vi "GUI Measurement setup.vi"(11 "Measurement properties":T3={"Measurement ID"=enum."1 signal, 1 ADC, 1 PJVS", "Description"="3 phase, 3 ADC, 1 PJVS", "Switching matrix M"=[], "Signal frequency  (Hz)"=50.0, "Maximal signal amplitude (V)"=0.0, "PRs (s)"=1.0, "PRe (s)"=10.0, "MRs (s)"=0.0, "MRe (s)"=0.0, "Set PJVS frequency (Hz)"=50.0, "PJVS reference voltages (1 period, V)"=[], "Requiested PJVS steps"=10, "Sampling f (Hz)"=0.0, "Trigger mode"=enum."Trigger every MX switch", "Timing matrix (periods)"=[], "Record length (multiples of M)"=1, "Calculated"={"Triggers to next path (line of sequence)"=[], "Record samples"=0, "Sample indexes of switches"=[], "PRs (samples)"=0, "PRe (samples)"=0, "MRs (samples)"=0, "MRe (samples)"=0, "Trigger frequency  (Hz)"=50.0, "Measurement druation (s)"=0.0, "Samples per step"=0.0, "QPMX Sequence"=[]}, "No of required digitizers"=0, "No of required transducers"=0, "Transducer correction files"=[], "Digitizer correction file"=path ""} {"Calculated"."Trigger frequency  (Hz)" format="%#_6p"; "Record length (multiples of M)" min=1 step=1; "PJVS reference voltages (1 period, V)" format="%.9g"; "MRe (s)" format="%#_4p"; "MRs (s)" format="%#_4p"; "PRe (s)" format="%#.4p"; "PRs (s)" format="%#_4p"}) -> (3 "Measurement properties out":T3={"Measurement ID"=enum."1 signal, 1 ADC, 1 PJVS", "Description"="3 phase, 3 ADC, 1 PJVS", "Switching matrix M"=[], "Signal frequency  (Hz)"=50.0, "Maximal signal amplitude (V)"=0.0, "PRs (s)"=1.0, "PRe (s)"=10.0, "MRs (s)"=0.0, "MRe (s)"=0.0, "Set PJVS frequency (Hz)"=50.0, "PJVS reference voltages (1 period, V)"=[], "Requiested PJVS steps"=10, "Sampling f (Hz)"=0.0, "Trigger mode"=enum."Trigger every MX switch", "Timing matrix (periods)"=[], "Record length (multiples of M)"=1, "Calculated"={"Triggers to next path (line of sequence)"=[], "Record samples"=0, "Sample indexes of switches"=[], "PRs (samples)"=0, "PRe (samples)"=0, "MRs (samples)"=0, "MRe (samples)"=0, "Trigger frequency  (Hz)"=50.0, "Measurement druation (s)"=0.0, "Samples per step"=0.0, "QPMX Sequence"=[]}, "No of required digitizers"=0, "No of required transducers"=0, "Transducer correction files"=[], "Digitizer correction file"=path ""} {"Calculated"."Trigger frequency  (Hz)" format="%#_6p"; "Record length (multiples of M)" min=1 step=1; "PJVS reference voltages (1 period, V)" format="%.9g"; "MRe (s)" format="%#_4p"; "MRs (s)" format="%#_4p"; "PRe (s)" format="%#.4p"; "PRs (s)" format="%#_4p"})   [LabVIEW 2020]
doc: "Use this template to build a producer/consumer design pattern with events to produce queue items. Use this design pattern instead of the User Interface Event Handler pattern for user interfaces when you want to execute code asynchronously in response to an event without slowing the user interface responsiveness."
uses:
  Measurement/Type definitions/Measuement properties.ctl
  Measurement/Type definitions/Measurement ID.ctl
  Measurement/Type definitions/Trigger mode.ctl
  <vilib>/Utility/error.llb/Error Cluster From Error Code.vi
  <vilib>/ErrorRing/Error Ring.xnode
  external libraries/varilib/varilib.lvlib
panel:
  in  "Digitizer correction file":path
  out "No of transducer corrections":u32=50 caption="Transducer corrections for           transducers."
  out "No of digitizer channels corrections":u32=50 caption="Corrections for           digitizer channels."
  in  "Transducer correction files":path[](array[path])
  out "required transducers":u32=50 caption="required."
  out "required digitizers":u32=50 caption="required."
  out "Connections image":picture
  out "Waveforms image":picture
  out "Samples per step":dbl
  out "Measurement druation (s)":dbl caption="Duration" format="%#_6p"
  in  "Maximal signal amplitude (V)":dbl caption="Maximal signal amplitude (at digitizer)"
  in  "Trigger mode":T1 caption="Mode"
  in  "Measurement setup ID":T2=enum."1 signal, 1 ADC, 1 PJVS" caption="Measurement scenario"
  out "Record samples":u32 format="%.0p"
  in  "Record length (multiples of M)":u32=1 min=1 step=1
  out "Trigger frequency  (Hz)":dbl=50.0 caption="Trigger frequency" format="%#_6p"
  in  "Sampling f (Hz)":dbl caption="Sampling frequency" format="%#_6p"
  in  "Requiested PJVS steps":u32=1 min=1 step=1
  in  "MRe (s)":dbl min=0.0 format="%#_4p"
  in  "MRs (s)":dbl min=0.0 format="%#_4p"
  in  "PRe (s)":dbl min=0.0 format="%#_4p"
  in  "PRs (s)":dbl min=0.0 format="%#_4p"
  in  "Signal frequency  (Hz)":dbl=50.0 caption="Signal frequency" format="%#_6p"
  out "Description":string
  out "gui_elements":refnum<vi>[](array[refnum])
  in  "save_and_quit":bool
  in  "cancel":bool
  # "Scenario"
  # "Signals"
  # "Hz"
  # "V"
  # "Sampling"
  # "Who will make\nnice pictures?\n\nconnection setup here"
  # "Hz"
  # "s"
  # "Trigger"
  # "Hz"
  # "PJVS"
  # "Who will make\nnice pictures?\n\nwaveforms here"
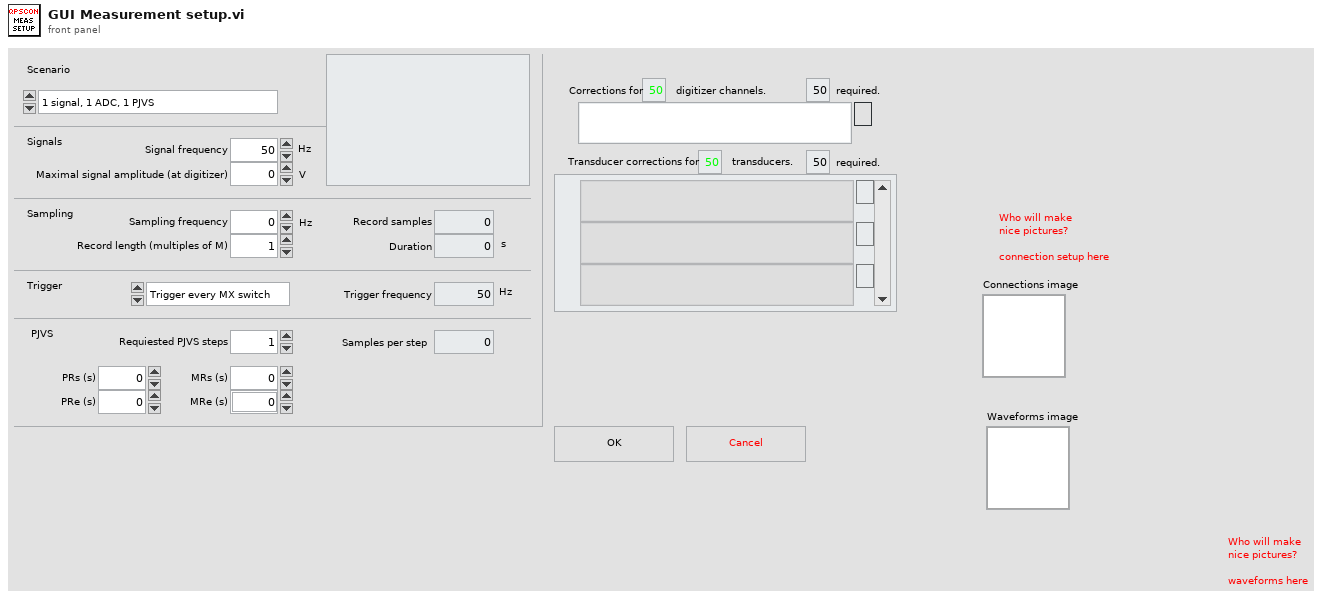
[diagram p1: front panel]
types:
  T1 = typedef "Trigger mode.ctl" = enum16{"Trigger every MX switch", "Trigger every sample"}
  T2 = typedef "Measurement ID.ctl" = enum16{"Manual setup", "1 signal, 1 ADC, 1 PJVS", "1 phase (U, I), 1 ADC, 1 PJVS", "1 phase (U, I), 2 ADC, 1 PJVS", "1 phase (U, I), 3 ADC, 1 PJVS", "3 phases (U1..3, I1..3), 3 ADC, 1 PJVS"}
  T3 = typedef "Measuement properties.ctl" = cluster{"Measurement ID":T2, "Description":string, "Switching matrix M":i32[][], "Signal frequency  (Hz)":dbl, "Maximal signal amplitude (V)":dbl, "PRs (s)":dbl, "PRe (s)":dbl, "MRs (s)":dbl, "MRe (s)":dbl, "Set PJVS frequency (Hz)":dbl, "PJVS reference voltages (1 period, V)":dbl[], "Requiested PJVS steps":u32, "Sampling f (Hz)":dbl, "Trigger mode":T1, "Timing matrix (periods)":i32[], "Record length (multiples of M)":u32, "Calculated":cluster{"Triggers to next path (line of sequence)":u32[], "Record samples":u32, "Sample indexes of switches":u32[], "PRs (samples)":i32, "PRe (samples)":i32, "MRs (samples)":i32, "MRe (samples)":i32, "Trigger frequency  (Hz)":dbl, "Measurement druation (s)":dbl, "Samples per step":dbl, "QPMX Sequence":bool[][]}, "No of required digitizers":u32, "No of required transducers":u32, "Transducer correction files":path[], "Digitizer correction file":path}
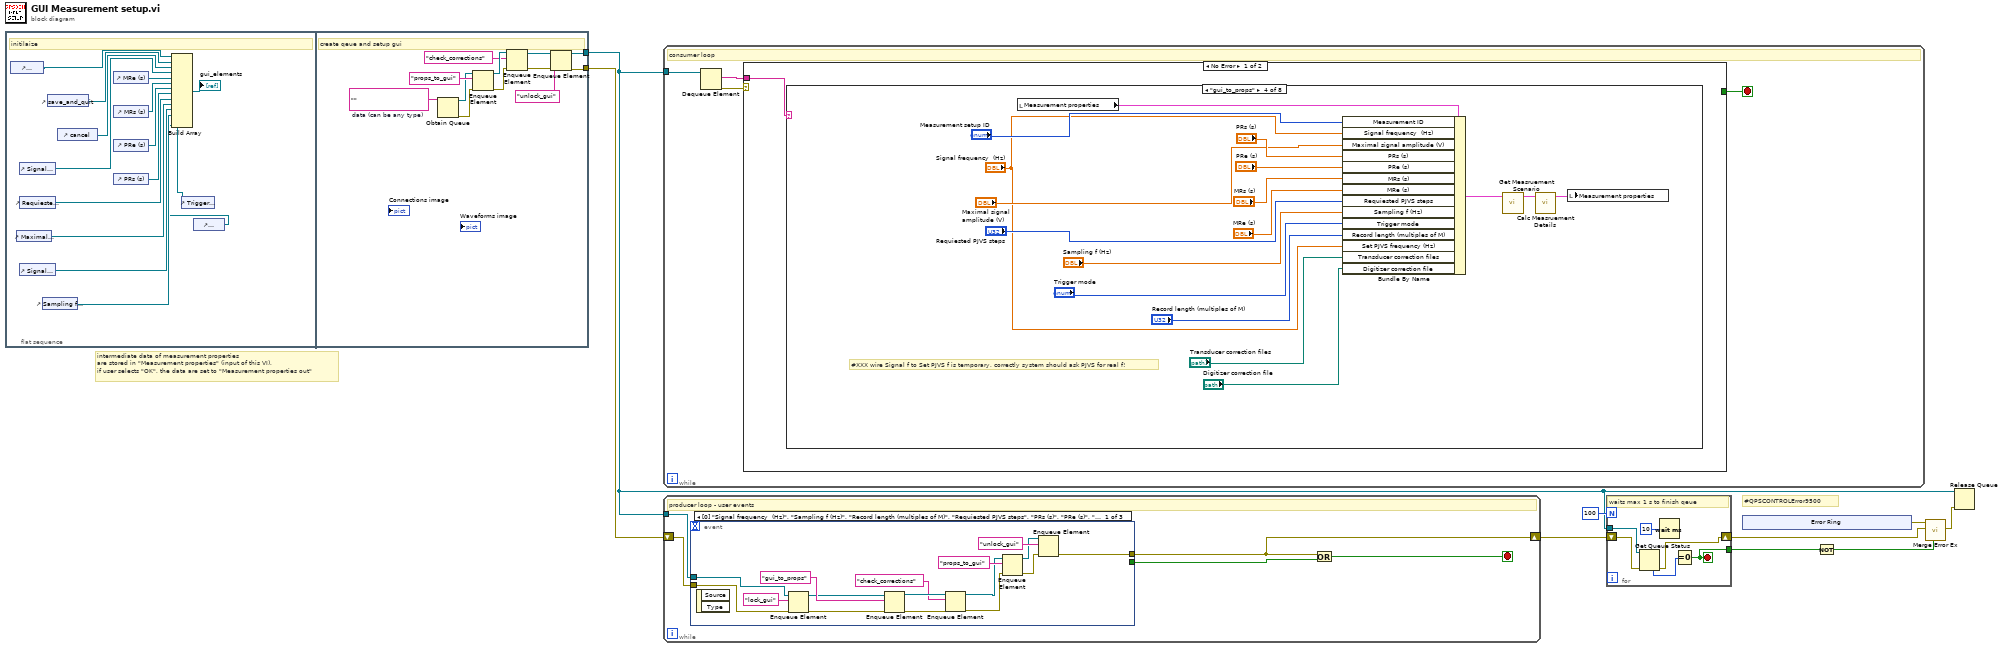
[diagram p0: block diagram]
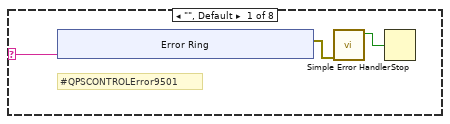
[diagram p2: hidden frame]
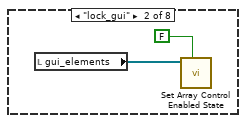
[diagram p3: hidden frame]
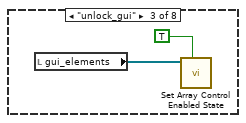
[diagram p4: hidden frame]
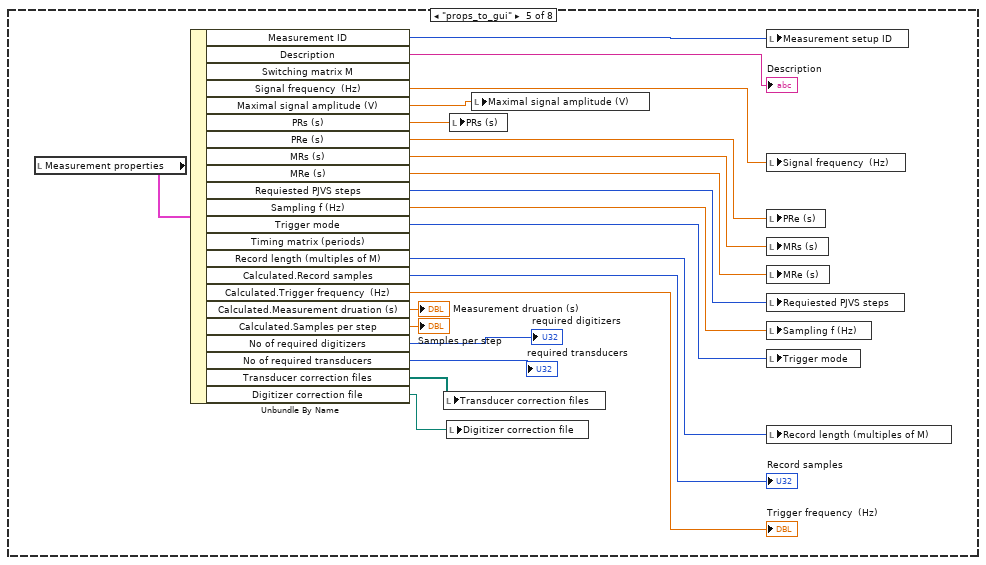
[diagram p5: hidden frame]
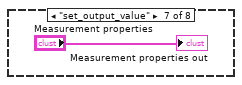
[diagram p7: hidden frame]
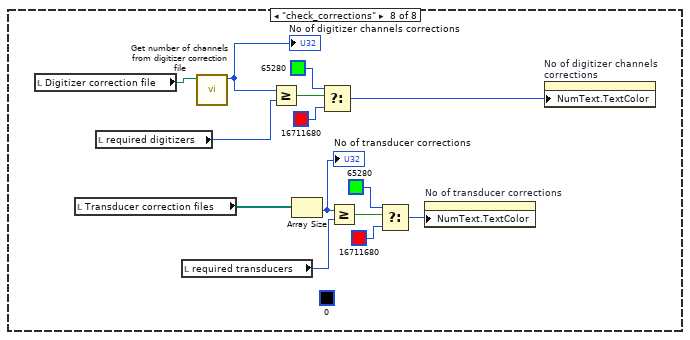
[diagram p8: hidden frame]
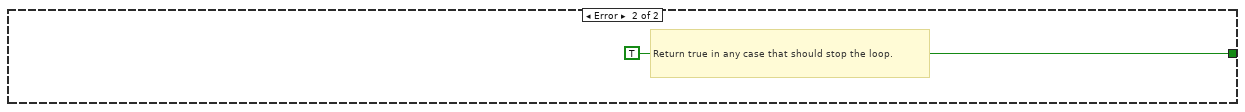
[diagram p9: hidden frame]
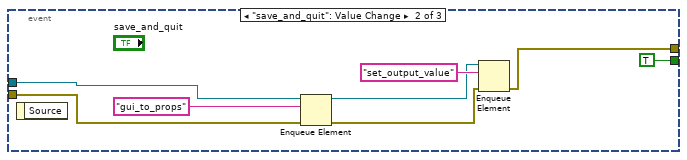
[diagram p10: hidden frame]
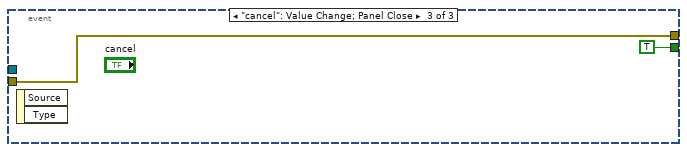
[diagram p11: hidden frame]
diagram:
  # "#QPSCONTROLError9500"
  # "intermediate data of measurement properties\nare stored in \"Measurement properties\" (input of this VI),\nif user selects \"OK\", the data are set to \"Measurement properties out\""
  n1 = flat-sequence {
    tunnel: [w27] -> w2
    tunnel: [w28] -> w1
    frame #0 {
      # "initilaize"
      n2 = control-ref of="Measurement setup ID"() -> (w13:refnum<vi>)
      n3 = control-ref of="Maximal signal amplitude (V)"() -> (w11:refnum<vi>)
      n4 = control-ref of="Signal frequency  (Hz)"() -> (w21:refnum<vi>)
      n5 = control-ref of="Requiested PJVS steps"() -> (w15:refnum<vi>)
      n6 = control-ref of="Signal frequency  (Hz)"() -> (w16:refnum<vi>)
      n7 = control-ref of="Sampling f (Hz)"() -> (w14:refnum<vi>)
      n8 = control-ref of="save_and_quit"() -> (w24:refnum<vi>)
      n9 = control-ref of="cancel"() -> (w23:refnum<vi>)
      n10 = control-ref of="MRe (s)"() -> (w20:refnum<vi>)
      n11 = control-ref of="MRs (s)"() -> (w19:refnum<vi>)
      n12 = control-ref of="PRe (s)"() -> (w18:refnum<vi>)
      n13 = control-ref of="PRs (s)"() -> (w17:refnum<vi>)
      n14 = control-ref of="Trigger mode"() -> (w12:refnum<vi>)
      n15 = control-ref of="Transducer correction files"() -> (w10:refnum<vi>)
      n16 = Build Array(w13, w24, w23, w21, w20, w19, w18, w17, w15, w11, w16, w14, w12, w10) -> (→"gui_elements":refnum<vi>[])
    }
    frame #1 {
      w32 = ""  # data (can be any type)
      # "create qeue and setup gui"
      n17 = Obtain Queue(element data type=w32) -> (queue out=w31:refnum<queue>, error out=w30:errorcluster)  [unwired: 4 in, 1 out]
      n18 = Enqueue Element(queue=w31, element="props_to_gui", error in (no error)=w30) -> (queue out=w36:refnum<queue>, error out=w35:errorcluster)  [unwired: 1 in, 1 out]
      n19 = Enqueue Element(queue=w36, element="check_corrections", error in (no error)=w35) -> (queue out=w26:refnum<queue>, error out=w29:errorcluster)  [unwired: 1 in, 1 out]
      n20 = Enqueue Element(queue=w26, element="unlock_gui", error in (no error)=w29) -> (queue out=w27:refnum<queue>, error out=w28:errorcluster)  [unwired: 1 in, 1 out]
    }
  }
  n21 = while {
    tunnel: w2 -> [w40]
    stop <- w37 stop-if-true
    # "consumer loop"
    n22 = Dequeue Element(queue=w40) -> (element=w38:string, error out=w39:errorcluster)  [unwired: 2 in, 2 out]
    n23 = case shown="No Error" w39 {
      tunnel: w38 -> [w41 _]
      tunnel: [_ TRUE] -> w37
      frame No Error {
        n24 = case shown="\"gui_to_props\"" w41 {
          selector: w41 -> [w42 _ _ _ _ _ _ _]
          frame "", Default {
            # "#QPSCONTROLError9501"
            n25 = xnode "Error Ring"("parameter 0"=w42) -> ("error out"=w44:errorcluster)
            n26 = call <vilib>:"Simple Error Handler.vi"("error in (no error)"=w44) -> ("error?"=w43:bool)  [unwired: 4 in, 4 out]
            n27 = Stop(stop? (T)=w43) -> ()
          }
          frame "lock_gui" {
            n28 = local read "gui_elements"() -> (w53:refnum<vi>[])
            n29 = call "Set Array Control Enabled State.vi"("enabled (T)"=FALSE, "reference array in"=w53) -> ()  [unwired: 8 in, 2 out]
          }
          frame "unlock_gui" {
            n30 = local read "gui_elements"() -> (w55:refnum<vi>[])
            n31 = call "Set Array Control Enabled State.vi"("enabled (T)"=TRUE, "reference array in"=w55) -> ()  [unwired: 8 in, 2 out]
          }
          frame "gui_to_props" {
            # "#XXX wire Signal f to Set PJVS f is temporary, correctly system should ask PJVS for real f!"
            n32 = local read "Measurement properties"() -> (w72:T3)
            n33 = Bundle By Name(cluster=w72, "Measurement ID"="Measurement setup ID", "Signal frequency  (Hz)"="Signal frequency  (Hz)", "Maximal signal amplitude (V)"="Maximal signal amplitude (V)", "PRs (s)"="PRs (s)", "PRe (s)"="PRe (s)", "MRs (s)"="MRs (s)", "MRe (s)"="MRe (s)", "Requiested PJVS steps"="Requiested PJVS steps", "Sampling f (Hz)"="Sampling f (Hz)", "Trigger mode"="Trigger mode", "Record length (multiples of M)"="Record length (multiples of M)", "Set PJVS frequency (Hz)"="Signal frequency  (Hz)", "Transducer correction files"="Transducer correction files", "Digitizer correction file"="Digitizer correction file") -> (w71:T3)
            n34 = call "Get Measruement Scenario.vi"("Measurement properties"=w71) -> ("Measurement properties out"=w70:T3)  [unwired: 10 in]
            n35 = call "Calc Measruement Details.vi"("Measurement properties"=w70) -> ("Measurement properties out"=w69:T3)  [unwired: 10 in]
            n36 = local write "Measurement properties"(w69) -> ()
          }
          frame "props_to_gui" {
            n37 = local read "Measurement properties"() -> (w86:T3)
            n38 = Unbundle By Name(w86) -> ("Measurement ID"=w93:T2, "Description"=→"Description":string, "Signal frequency  (Hz)"=w91:dbl, "Maximal signal amplitude (V)"=w79:dbl, "PRs (s)"=w90:dbl, "PRe (s)"=w89:dbl, "MRs (s)"=w88:dbl, "MRe (s)"=w87:dbl, "Requiested PJVS steps"=w85:u32, "Sampling f (Hz)"=w84:dbl, "Trigger mode"=w83:T1, "Record length (multiples of M)"=w82:u32, "Calculated.Record samples"=→"Record samples":u32, "Calculated.Trigger frequency  (Hz)"=→"Trigger frequency  (Hz)":dbl, "Calculated.Measurement druation (s)"=→"Measurement druation (s)":dbl, "Calculated.Samples per step"=→"Samples per step":dbl, "No of required digitizers"=→"required digitizers":u32, "No of required transducers"=→"required transducers":u32, "Transducer correction files"=w74:path[], "Digitizer correction file"=w73:path)  [unwired: 2 out]
            n39 = local write "Transducer correction files"(w74) -> ()
            n40 = local write "Digitizer correction file"(w73) -> ()
            n41 = local write "PRs (s)"(w90) -> ()
            n42 = local write "Maximal signal amplitude (V)"(w79) -> ()
            n43 = local write "Measurement setup ID"(w93) -> ()
            n44 = local write "Signal frequency  (Hz)"(w91) -> ()
            n45 = local write "PRe (s)"(w89) -> ()
            n46 = local write "MRs (s)"(w88) -> ()
            n47 = local write "MRe (s)"(w87) -> ()
            n48 = local write "Requiested PJVS steps"(w85) -> ()
            n49 = local write "Sampling f (Hz)"(w84) -> ()
            n50 = local write "Trigger mode"(w83) -> ()
            n51 = local write "Record length (multiples of M)"(w82) -> ()
          }
          frame "ask_PJVS" {
            # "#XXX here will be:  init PJVS, ask for PJVS values, close PJVS."
          }
          frame "set_output_value" {
            "Measurement properties out" <- "Measurement properties"
          }
          frame "check_corrections" {
            (unwired) u32 0 ("Numeric Text.Text Colors:Text Color")
            n52 = local read "Digitizer correction file"() -> (w96:path)
            n53 = local read "Transducer correction files"() -> (w108:path[])
            n54 = local read "required digitizers"() -> (w98:u32)
            n55 = local read "required transducers"() -> (w107:u32)
            n56 = call "Get number of channels from digitizer correction file.vi"("Correction file path"=w96) -> ("Number of channels"=w95:u32)  [unwired: 10 in]
            "No of digitizer channels corrections" <- w95
            n57 = Greater Or Equal?(x=w95, y=w98) -> (x >= y?=w99:bool)
            n58 = Array Size(array=w108) -> (size(s)=w102:i32)
            "No of transducer corrections" <- w102
            n59 = Select(t=u32 65280 ("Numeric Text.Text Colors:Text Color"), s=w99, f=u32 16711680 ("Numeric Text.Text Colors:Text Color")) -> (s? t:f=w97:u32)
            n60 = Greater Or Equal?(x=w102, y=w107) -> (x >= y?=w106:bool)
            n61 = Select(t=u32 65280 ("Numeric Text.Text Colors:Text Color"), s=w106, f=u32 16711680 ("Numeric Text.Text Colors:Text Color")) -> (s? t:f=w103:u32)
            n62 = property on="No of transducer corrections" class="DigNum (strict)"("NumText.TextColor"=w103) -> ()  [unwired: 2 in, 2 out]
            n63 = property on="No of digitizer channels corrections" class="DigNum (strict)"("NumText.TextColor"=w97) -> ()  [unwired: 2 in, 2 out]
          }
        }
      }
      frame Error {
        # "Return true in any case that should stop the loop."
      }
    }
  }
  n64 = while {
    shift-right: [w110] -> w5
    shift-left: w1 -> [w113]
    tunnel: w2 -> [w114]
    stop <- w111 stop-if-true
    # "producer loop - user events"
    n65 = event shown="[0] \"Signal frequency  (Hz)\", \"Sampling f (Hz)\", \"Record length (multiples of M)\", \"Requiested PJVS steps\", \"PRs (s)\", \"PRe (s)\", \"MRs (s)\", \"MRe (s)\", \"Measurement setup ID\", \"Trigger mode\", \"Maximal signal amplitude (V)\", \"Transducer correction files\", \"Digitizer correction file\": Value Change" {
      selector: _ -> [_ _ _]
      dyn-events: _ -> [_ _ _]
      timeout: _ -> [_ _ _]
      tunnel: w114 -> [w126 w135 _]
      tunnel: w113 -> [w127 w132 w140]
      tunnel: [w129 w131 w140] -> w110
      tunnel: [_ TRUE ("cancel") TRUE ("cancel")] -> w112
      event "Signal frequency  (Hz)", "Sampling f (Hz)", "Record length (multiples of M)", "Requiested PJVS steps", "PRs (s)", "PRe (s)", "MRs (s)", "MRe (s)", "Maximal signal amplitude (V)", "Transducer correction files", "Digitizer correction file": Value Change {
        n66 = event-data() -> ()  [unwired: 1 in, 2 out]
        n67 = Enqueue Element(queue=w126, element="lock_gui", error in (no error)=w127) -> (queue out=w124:refnum<queue>, error out=w123:errorcluster)  [unwired: 1 in, 1 out]
        n68 = Enqueue Element(queue=w124, element="gui_to_props", error in (no error)=w123) -> (queue out=w116:refnum<queue>, error out=w119:errorcluster)  [unwired: 1 in, 1 out]
        n69 = Enqueue Element(queue=w116, element="check_corrections", error in (no error)=w119) -> (queue out=w117:refnum<queue>, error out=w118:errorcluster)  [unwired: 1 in, 1 out]
        n70 = Enqueue Element(queue=w117, element="props_to_gui", error in (no error)=w118) -> (queue out=w120:refnum<queue>, error out=w121:errorcluster)  [unwired: 1 in, 1 out]
        n71 = Enqueue Element(queue=w120, element="unlock_gui", error in (no error)=w121) -> (error out=w129:errorcluster)  [unwired: 1 in, 2 out]
      }
      event "save_and_quit": Value Change {
        n72 = event-data() -> ()  [unwired: 1 in, 1 out]
        n73 = Enqueue Element(queue=w135, element="gui_to_props", error in (no error)=w132) -> (queue out=w134:refnum<queue>, error out=w133:errorcluster)  [unwired: 1 in, 1 out]
        n74 = Enqueue Element(queue=w134, element="set_output_value", error in (no error)=w133) -> (error out=w131:errorcluster)  [unwired: 1 in, 2 out]
      }
      event "cancel": Value Change; Panel Close {
        n75 = event-data() -> ()  [unwired: 1 in, 2 out]
      }
    }
    n76 = Or(x=w110, y=w112) -> (x .or. y?=w111:bool)
  }
  n77 = for {
    N: 100 -> [_]
    tunnel: w2 -> [w146]
    shift-right: [w144] -> w6
    shift-left: w5 -> [w145]
    tunnel: [w141] -> w3
    stop <- w141 stop-if-true
    # "waits max 1 s to finish qeue"
    n78 = Get Queue Status(queue=w146, error in (no error)=w145) -> (error out=w144:errorcluster, # elements in queue=w142:i32)  [unwired: 1 in, 6 out]
    n79 = Wait (ms)(milliseconds to wait=u32 10) -> ()  [unwired: 1 out]
    n80 = Equal To 0?(x=w142) -> (x = 0?=w141:bool)
  }
  n81 = xnode "Error Ring"() -> ("error out"=w7:errorcluster)
  n82 = Not(x=w3) -> (.not. x?=w8:bool)
  n83 = call "Merge Error Ex.vi"("Is error? (False)"=w8, "main error in (no error)"=w6, "second error in"=w7) -> ("error out"=w4:errorcluster)  [unwired: 8 in]
  n84 = Release Queue(queue=w2, error in (no error)=w4) -> ()  [unwired: 1 in, 3 out]
